vi "Resume.vi"(6 "nargs":i32, 8 "error in (no error)":errorcluster, 11 "Lua in":refnum<data-value>) -> (0 "error out":errorcluster, 1 "done?":bool, 3 "Lua out":refnum<data-value>, 4 "nresults":i32)   [LabVIEW 2020, in "Lua for LabVIEW.lvlib" / "Lua.lvclass"]
doc: "Starts and resumes a coroutine in the given thread L.\n\nTo start a coroutine, you push onto the thread stack the main function plus any arguments; then you call lua_resume, with nargs being the number of arguments. This call returns when the coroutine suspends or finishes its execution. When it returns, the stack contains all values passed to lua_yield, or all values returned by the body function. lua_resume returns LUA_YIELD if the coroutine yields, LUA_OK if the coroutine finishes its execution without errors, or an error code in case of errors (see lua_pcall).\n\nIn case of errors, the stack is not unwound, so you can use the debug API over it. The error object is on the top of the stack.\n\nTo resume a coroutine, you remove any results from the last lua_yield, put on its stack only the values to be passed as results from yield, and then call lua_resume.\n\nThe parameter from represents the coroutine that is resuming L. If there is no such coroutine, this parameter can be NULL."
uses:
  Lua.lvclass
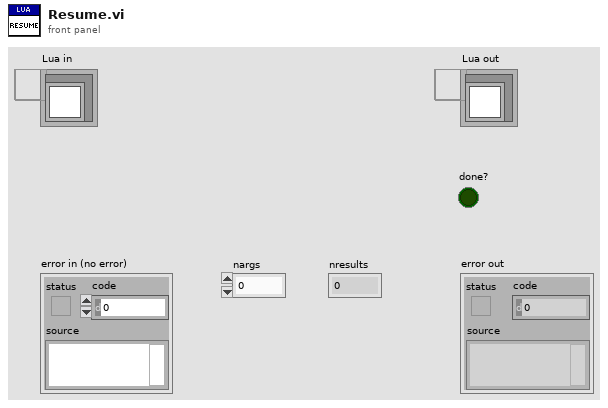
[diagram p1: front panel]
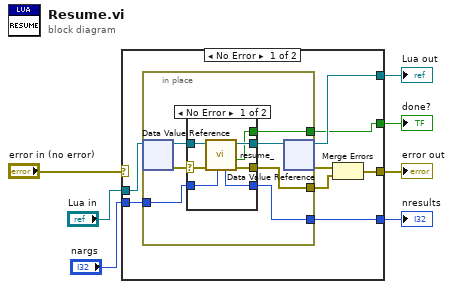
[diagram p0: block diagram]
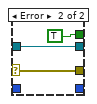
[diagram p2: hidden frame]
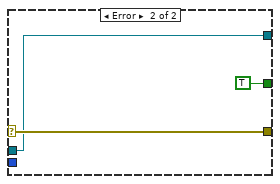
[diagram p3: hidden frame]
diagram:
  n1 = case shown="No Error" "error in (no error)" {
    selector: "error in (no error)" -> [_ w35]
    tunnel: [w13 w35] -> w6
    tunnel: [w11 w34] -> w4
    tunnel: "Lua in" -> [w15 w34]
    tunnel: "nargs" -> [w10 _]
    tunnel: [w9 TRUE ("done?")] -> w2
    tunnel: [w8 _] -> w1
    frame No Error {
      n2 = in-place {
        in-place-border: [w19] -> w12
        in-place-border: w10 -> [w18]
        in-place-border: [w17] -> w9
        in-place-border: [w16] -> w8
        n3 = in-place-dvr #1(w15) -> (w22:refnum<class "Lua.lvclass">, w20:errorcluster)
        n4 = case shown="No Error" w20 {
          selector: w20 -> [w23 w32]
          tunnel: w22 -> [w29 w31]
          tunnel: [w28 w31] -> w21
          tunnel: [w27 w32] -> w19
          tunnel: w18 -> [w24 _]
          tunnel: [w26 TRUE ("done?")] -> w17
          tunnel: [w25 _] -> w16
          frame No Error {
            n5 = call-dynamic "resume_.vi"("nargs"=w24, "error in (no error)"=w23, "Lua in"=w29) -> ("error out"=w27:errorcluster, "done?"=w26:bool, "Lua out"=w28:refnum<class "Lua.lvclass">, "nresults"=w25:i32)  [unwired: 5 in]
          }
          frame Error {
          }
        }
        n6 = in-place-dvr #1(w21) -> (w11:refnum<data-value>, w14:errorcluster)
      }
      n7 = Merge Errors(w14, w12) -> (w13:errorcluster)
    }
    frame Error {
    }
  }
  "error out" <- w6
  "Lua out" <- w4
  "nresults" <- w1
  "done?" <- w2
